vi "[FGV] Camera Settings.vi"(6 "CamSession":T1[](array[typedef]), 7 "Action":T3(ring), 8 "error in (no error)":errorcluster, 9 "SeqOn":bool, 10 "Value":u16, 11 "Image In":T2) -> (0 "error out":errorcluster, 2 "Camera Interface Name":T1[](array[typedef]), 3 "Image Out":T2)   [LabVIEW 2019]
uses:
  <vilib>/userdefined/High Color/IMAQdx.ctl
  <vilib>/vision/Image Controls.llb/IMAQ Image.ctl
  <vilib>/vision/driver/NI_Vision_Acquisition_Software.lvlib
  <resource>/objmgr/imaqdx.rc
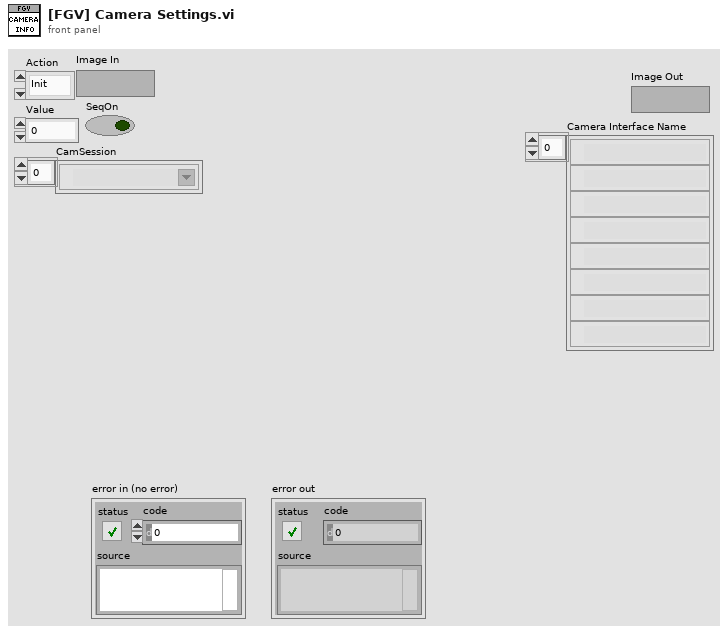
[diagram p1: front panel]
types:
  T1 = typedef "IMAQdx.ctl" = refnum<k21>
  T2 = typedef "IMAQ Image.ctl" = refnum<image>
  T3 = enum16{"Init", "Grab", "Get All", "Close", "Set Camera"}
  T4 = cluster{"Type":u32, "Version":u32, "Flags":u32, "SerialNumberHigh":u32, "SerialNumberLow":u32, "BusType":u32, "InterfaceName":string, "VendorName":string, "ModelName":string, "CameraFileName":string, "CameraAttributeURL":string}[]
  T5 = typedef "Image Type" = u32
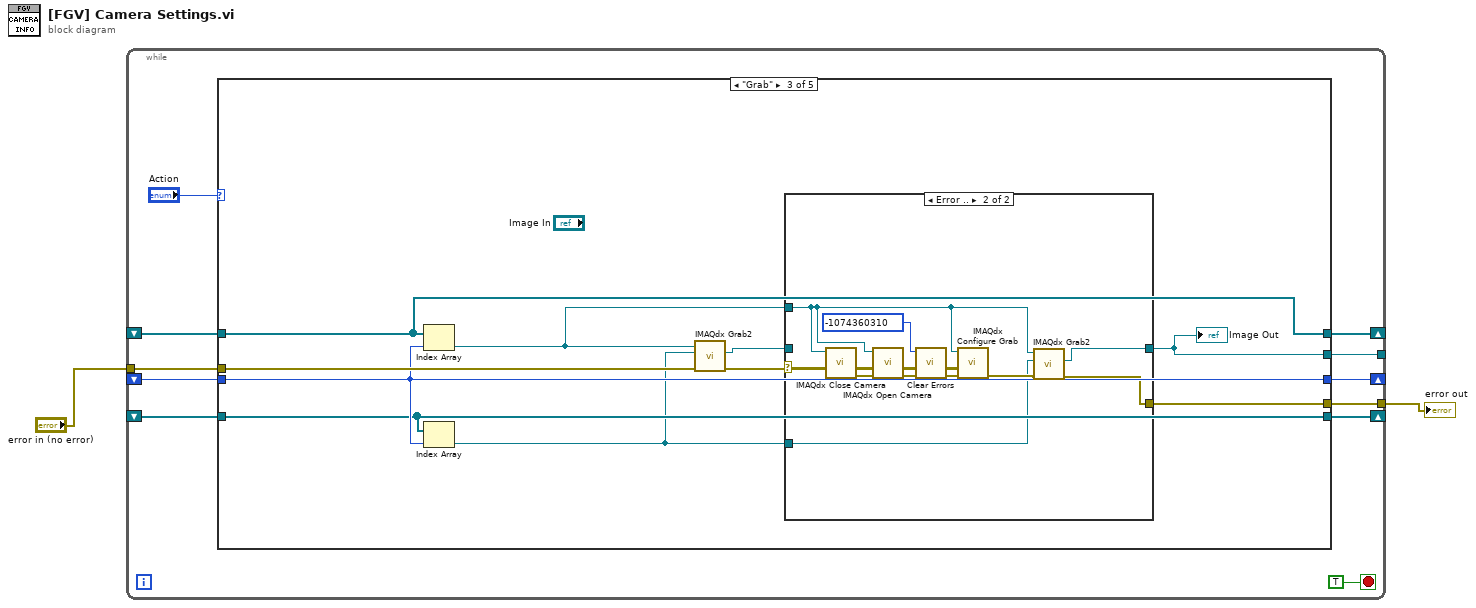
[diagram p0: block diagram]
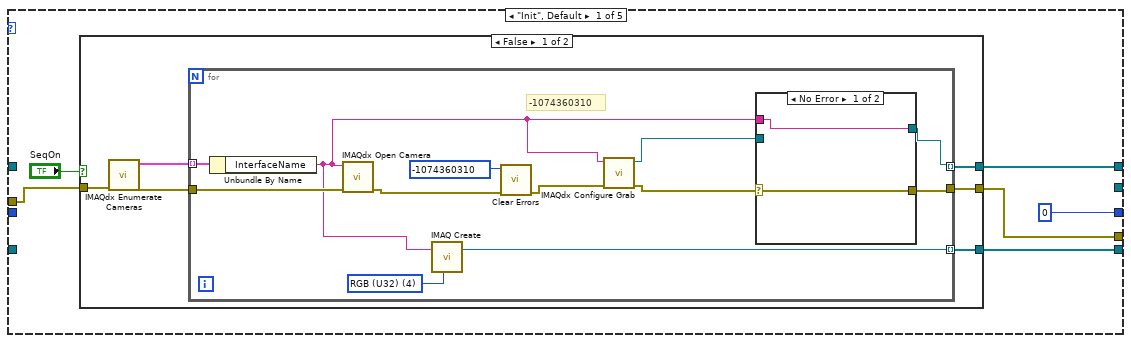
[diagram p2: hidden frame]
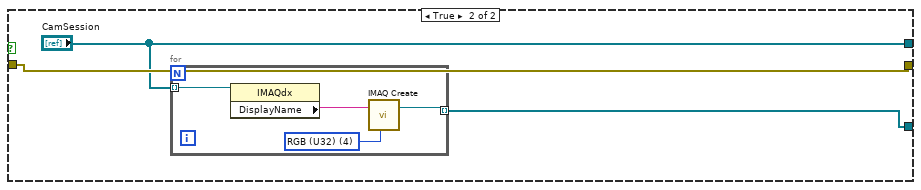
[diagram p4: hidden frame]
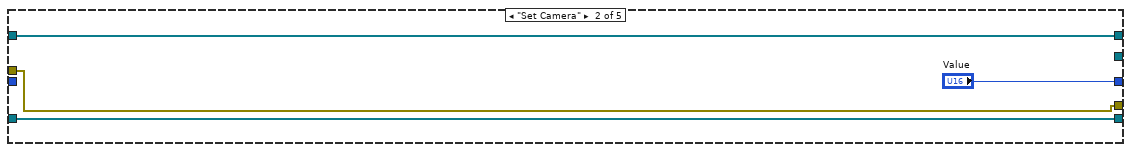
[diagram p5: hidden frame]
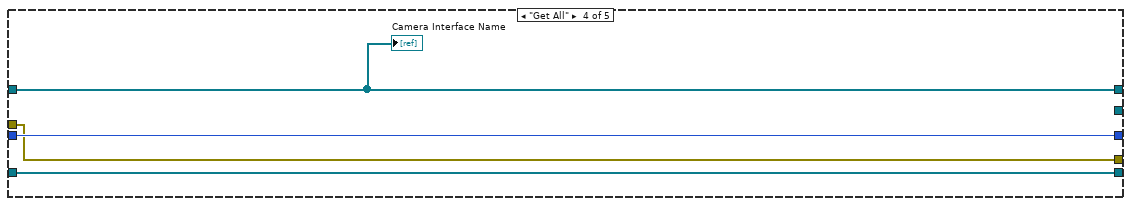
[diagram p7: hidden frame]
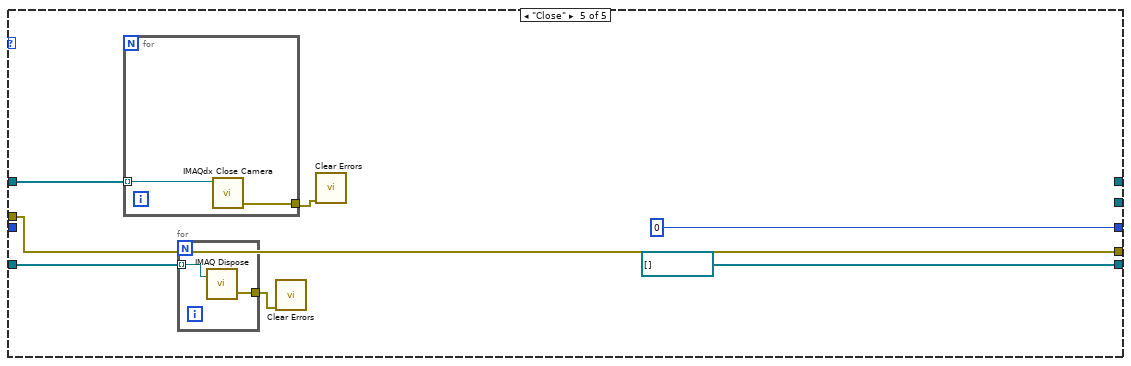
[diagram p8: hidden frame]
diagram:
  n1 = while {
    shift-right: [w11] -> _
    shift-left: _ -> [w10]
    tunnel: [w9] -> _
    shift-right: [w7] -> _
    shift-left: _ -> [w8]
    tunnel: [w6] -> w2
    tunnel: "error in (no error)" -> [w5]
    shift-right: [w4] -> _
    shift-left: _ -> [w3]
    stop <- TRUE stop-if-true
    n2 = case shown="\"Grab\"" "Action" {
      tunnel: [w19 w52 w62 w77 _] -> w11
      tunnel: w10 -> [_ w52 w62 w77 w84]
      tunnel: [_ _ w55 _ _] -> w9
      tunnel: w8 -> [_ _ w60 w76 _]
      tunnel: [u16 0 "Value" w60 w76 u16 0] -> w7
      tunnel: [w16 w50 w57 w75 w82] -> w6
      tunnel: w5 -> [w17 w50 w61 w75 w82]
      tunnel: [w14 w49 w59 w74 T2[] []] -> w4
      tunnel: w3 -> [_ w49 w59 w74 w80]
      frame "Init", Default {
        n3 = case shown="False" "SeqOn" {
          tunnel: [w25 "CamSession"] -> w19
          tunnel: w17 -> [w22 w44]
          tunnel: [w21 w44] -> w16
          tunnel: [w20 w42] -> w14
          frame False {
            n4 = call <vilib>:"IMAQdx Enumerate Cameras.vi"("error in"=w22) -> ("error out"=w23:errorcluster, "Camera Information Array"=w24:T4)  [unwired: 9 in]
            n5 = for {
              tunnel: w24 -> [w37] mode=indexing
              tunnel: [w32] -> w25 mode=indexing
              tunnel: w23 -> [w36]
              tunnel: [w31] -> w21
              tunnel: [w34] -> w20 mode=indexing
              w35 = T5 4 items=["Grayscale (U8)", "Grayscale (I16)", "Grayscale (SGL)", "Complex (CSG)", "RGB (U32)", "HSL (U32)", "RGB (U64)", "Grayscale (U16)"] ("Image Type")
              # "-1074360310"
              n6 = Unbundle By Name(w37) -> ("InterfaceName"=w26:string)
              n7 = call <vilib>:"IMAQdx Open Camera.vi"("error in"=w36, "Session In"=w26) -> ("error out"=w29:errorcluster)  [unwired: 1 in, 8 out]
              n8 = call "IMAQ Create"("Image Name"=w26, "Image Type"=w35) -> ("New Image"=w34:T2)  [unwired: 3 in, 1 out]
              n9 = call <vilib>:"Clear Errors.vi"("error in (no error)"=w29, "specific error code to clear (0: all)"=-1074360310 ("error code (0)")) -> ("error out"=w28:errorcluster)  [unwired: 4 in, 1 out]
              n10 = call <vilib>:"IMAQdx Configure Grab.vi"("error in"=w28, "Session In"=w26) -> ("error out"=w27:errorcluster, "Session Out"=w30:T1)  [unwired: 8 in]
              n11 = case shown="No Error" w27 {
                selector: w27 -> [w39 w40]
                tunnel: [w38 w41] -> w32
                tunnel: w30 -> [_ w41]
                tunnel: [w39 w40] -> w31
                tunnel: w26 -> [w38 _]
                frame No Error {
                }
                frame Error {
                }
              }
            }
          }
          frame True {
            n12 = for {
              tunnel: "CamSession" -> [w48] mode=indexing
              tunnel: [w45] -> w42 mode=indexing
              w47 = T5 4 items=["Grayscale (U8)", "Grayscale (I16)", "Grayscale (SGL)", "Complex (CSG)", "RGB (U32)", "HSL (U32)", "RGB (U64)", "Grayscale (U16)"] ("Image Type")
              n13 = property class="IMAQdx"(reference=w48) -> ("DisplayName"=w46:string)  [unwired: 1 in, 2 out]
              n14 = call "IMAQ Create"("Image Name"=w46, "Image Type"=w47) -> ("New Image"=w45:T2)  [unwired: 3 in, 1 out]
            }
          }
        }
      }
      frame "Set Camera" {
      }
      frame "Grab" {
        n15 = Index Array(array=w62, index=w60) -> (element=w54:T1)
        n16 = Index Array(array=w59, index=w60) -> (element=w53:T2)
        n17 = call <vilib>:"IMAQdx Grab2.vi"("error in"=w61, "Image In"=w53, "Session In"=w54) -> ("error out"=w58:errorcluster, "Image Out"=w56:T2)  [unwired: 5 in, 2 out]
        n18 = case shown="Error .." w58 {
          selector: w58 -> [w63 _]
          tunnel: [w63 w68] -> w57
          tunnel: w56 -> [w64 _]
          tunnel: [w64 w67] -> w55
          tunnel: w54 -> [_ w66]
          tunnel: w53 -> [_ w65]
          frame No Error {
          }
          frame Error {
            n19 = call <vilib>:"IMAQdx Close Camera.vi"("Session In"=w66) -> ("error out"=w70:errorcluster)  [unwired: 10 in]
            n20 = call <vilib>:"IMAQdx Open Camera.vi"("error in"=w70, "Session In"=w66) -> ("error out"=w73:errorcluster)  [unwired: 1 in, 8 out]
            n21 = call <vilib>:"Clear Errors.vi"("error in (no error)"=w73, "specific error code to clear (0: all)"=-1074360310 ("error code (0)")) -> ("error out"=w72:errorcluster)  [unwired: 4 in, 1 out]
            n22 = call <vilib>:"IMAQdx Configure Grab.vi"("error in"=w72, "Session In"=w66) -> ("error out"=w69:errorcluster)  [unwired: 8 in, 1 out]
            n23 = call <vilib>:"IMAQdx Grab2.vi"("error in"=w69, "Image In"=w65, "Session In"=w66) -> ("error out"=w68:errorcluster, "Image Out"=w67:T2)  [unwired: 5 in, 2 out]
          }
        }
        "Image Out" <- w55
      }
      frame "Get All" {
        "Camera Interface Name" <- w77
      }
      frame "Close" {
        n24 = for {
          tunnel: w84 -> [w88] mode=indexing
          tunnel: [w87] -> w81
          n25 = call <vilib>:"IMAQdx Close Camera.vi"("Session In"=w88) -> ("error out"=w87:errorcluster)  [unwired: 1 in, 9 out]
        }
        n26 = for {
          tunnel: w80 -> [w86] mode=indexing
          tunnel: [w85] -> w79
          n27 = call "IMAQ Dispose"("Image"=w86) -> ("error out"=w85:errorcluster)  [unwired: 5 in]
        }
        n28 = call <vilib>:"Clear Errors.vi"("error in (no error)"=w79) -> ()  [unwired: 5 in, 2 out]
        n29 = call <vilib>:"Clear Errors.vi"("error in (no error)"=w81) -> ()  [unwired: 5 in, 2 out]
      }
    }
  }
  "error out" <- w2
